vi "InAndOutGB.vi"() -> ()   [LabVIEW 2019]
panel:
  in  "Card_0":bool[](array[boolean])
  in  "Card_1":bool[](array[boolean])
  in  "Card_6":bool[](array[boolean])
  in  "Card_5":bool[](array[boolean])
  in  "Card_4":bool[](array[boolean])
  in  "Card_3":bool[](array[boolean])
  in  "Card_2":bool[](array[boolean])
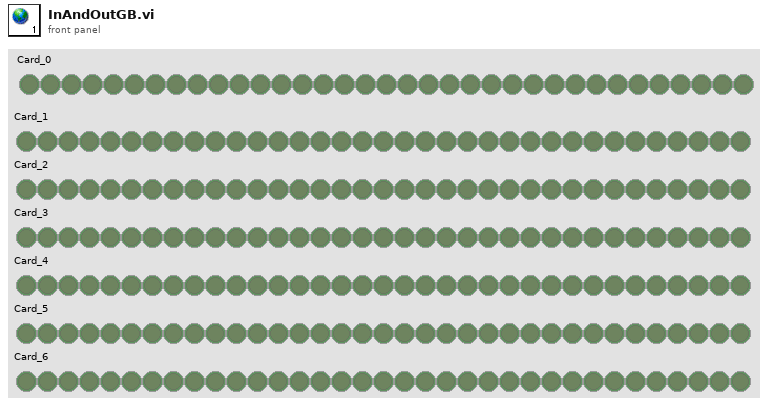
[diagram p1: front panel]
diagram:
